vi "Callback - Subscribed names.vi"(8 "error in (no error)":errorcluster, 10 "Subscribed names":string[](array[string]), 11 "BluePlotHandle in":refnum<class "RocketPlotHandle.lvclass">) -> (0 "error out":errorcluster, 3 "BluePlotHandle out":refnum<class "RocketPlotHandle.lvclass">)   [LabVIEW 2021, in "RocketPlotHandle.lvclass"]
uses:
  RocketPlotHandle.lvclass
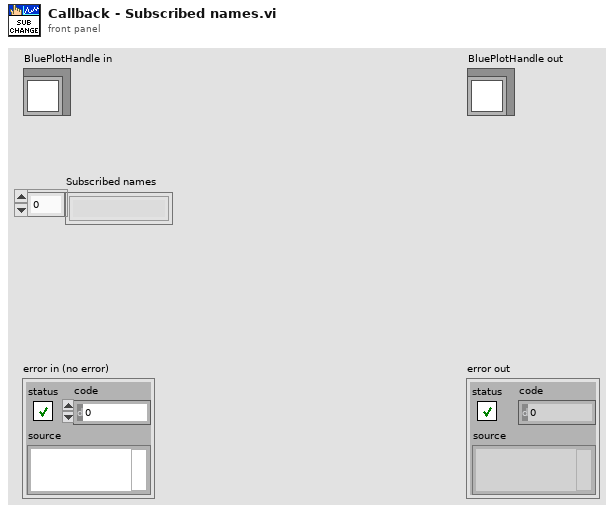
[diagram p1: front panel]
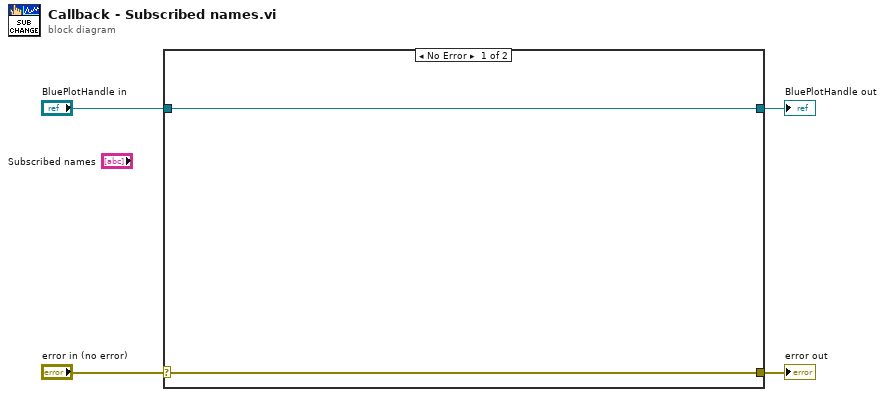
[diagram p0: block diagram]
diagram:
  n1 = case shown="No Error" "error in (no error)" {
    selector: "error in (no error)" -> [w5 w8]
    tunnel: [w5 w8] -> w3
    tunnel: [w6 w7] -> w1
    tunnel: "BluePlotHandle in" -> [w6 w7]
    frame No Error {
    }
    frame Error {
    }
  }
  "error out" <- w3
  "BluePlotHandle out" <- w1
